vi "DSF.Engine.Runtime.Framework.Get Plugin Runtimes.vi"(11 "Framework Runtime in":refnum<class "DSF.Engine.Runtime.Framework.lvclass">) -> (2 "Plugin Runtimes":refnum<class "DSF.Engine.Plugin.Runtime.lvclass">[](array[class]), 3 "Framework Runtime out":refnum<class "DSF.Engine.Runtime.Framework.lvclass">)   [LabVIEW 2016, in "DSF.Engine.lvlib" / "DSF.Engine.Runtime.Framework.lvclass"]
uses:
  DSF.Engine.Runtime.Framework.lvclass
  Plugin/DSF.Engine.Plugin.Runtime.lvclass
  DSF.Engine.Runtime.Framework.lvclass/DSF.Engine.Runtime.Framework.ctl
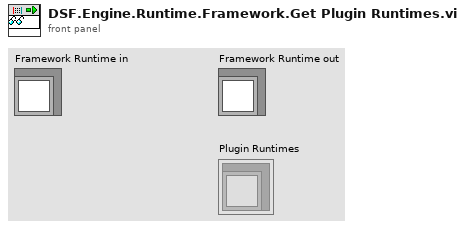
[diagram p1: front panel]
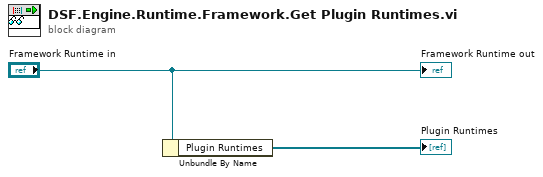
[diagram p0: block diagram]
diagram:
  n1 = Unbundle By Name("Framework Runtime in") -> ("Plugin Runtimes"=→"Plugin Runtimes":refnum<class "DSF.Engine.Plugin.Runtime.lvclass">[])
  "Framework Runtime out" <- "Framework Runtime in"
